vi "JSR SetTrig.vi"(8 "error in (no error)":errorcluster, 10 "JSR Trigger Settings":T1 {"PRF (Hz)" items=["100 Hz"=0.1, "200 Hz"=0.2, "400 Hz"=0.4, "600 Hz"=0.6, "800 Hz"=0.8, "1000 Hz"=1.0, "1250 Hz"=1.25, "1500 Hz"=1.5, "1750 Hz"=1.75, "2000 Hz"=2.0, "2500 Hz"=2.5, "3000 Hz"=3.0, "3500 Hz"=3.5, "4000 Hz"=4.0, "4500 Hz"=4.5, "5000 Hz"=5.0]; "Trigger Source" items=["Internal", "External"]; "External Trigger Limit" items=["No Limit", "5 kHz"]}, 11 "VISA Refnum in":refnum<visa-resource-name>) -> (0 "error out":errorcluster, 3 "VISA Refnum out":refnum<visa-resource-name>)   [LabVIEW 2022 SP3]
uses:
  Controls/JSR Trigger.ctl
  Controls/Trig Limit.ctl
  Controls/Trig Source.ctl
  Controls/PRF.ctl
  PulserGlobals.vi
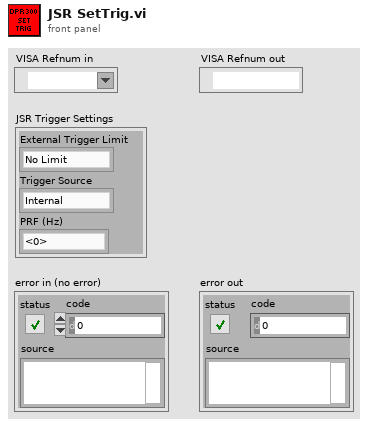
[diagram p1: front panel]
types:
  T1 = typedef "JSR Trigger.ctl" = cluster{"External Trigger Limit":T2, "Trigger Source":T3, "PRF (Hz)":T4}
  T2 = typedef "Trig Limit.ctl" = i8
  T3 = typedef "Trig Source.ctl" = i8
  T4 = typedef "PRF.ctl" = dbl
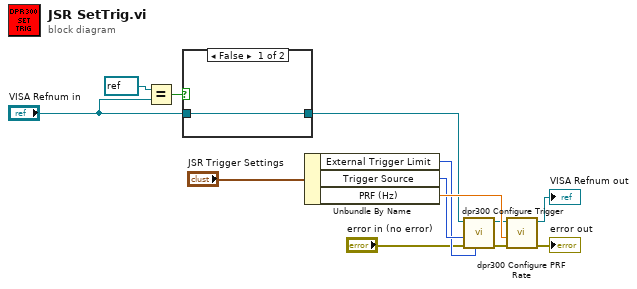
[diagram p0: block diagram]
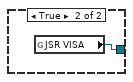
[diagram p2: hidden frame]
diagram:
  n1 = Equal?(x=refnum<visa-resource-name> refnum, y="VISA Refnum in") -> (x = y?=w3:bool)
  n2 = case shown="False" w3 {
    tunnel: [w14 w15] -> w1
    tunnel: "VISA Refnum in" -> [w14 _]
    frame False {
    }
    frame True {
      n3 = global read "PulserGlobals.vi" "JSR VISA"() -> (w15:refnum<visa-resource-name>)
    }
  }
  n4 = Unbundle By Name("JSR Trigger Settings") -> ("External Trigger Limit"=w11:T2, "Trigger Source"=w12:T3, "PRF (Hz)"=w13:T4)
  n5 = call <instrlib>:"dpr300 Configure Trigger.vi"("External Trigger Limit (0: No Limit)"=w11, "error in (no error)"="error in (no error)", "Trigger Source (0: Internal)"=w12, "VISA resource name"=w1) -> ("error out"=w9:errorcluster, "VISA resource name out"=w6:refnum<visa-resource-name>)  [unwired: 6 in]
  n6 = call <instrlib>:"dpr300 Configure PRF Rate.vi"("error in (no error)"=w9, "PRF Rate (7: 1500 Hz)"=w13, "VISA resource name"=w6) -> ("error out"=→"error out":errorcluster, "VISA resource name out"=→"VISA Refnum out":refnum<visa-resource-name>)  [unwired: 7 in]
